vi "initial.vi"(8 "error in (no error)":errorcluster, 10 "Path":path, 11 "CSV in":refnum<class "CSV.lvclass">) -> (0 "error out":errorcluster, 3 "CSV out":refnum<class "CSV.lvclass">)   [LabVIEW 2014, in "CSV.lvclass"]
uses:
  CSV.lvclass
  CSV.lvclass/CSV.ctl
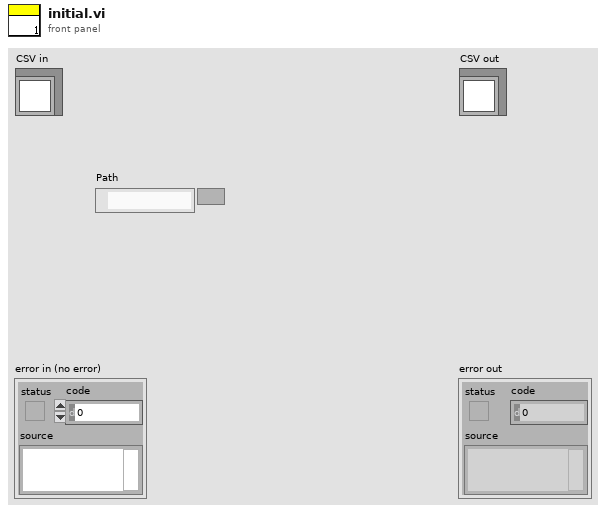
[diagram p1: front panel]
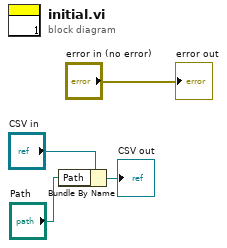
[diagram p0: block diagram]
diagram:
  n1 = Bundle By Name(cluster="CSV in", "Path"="Path") -> (→"CSV out":refnum<class "CSV.lvclass">)
  "error out" <- "error in (no error)"
